vi "test_ResolveService_WithNewClusterId_RetriesAndSucceeds.vi"(8 "error in":errorcluster) -> (0 "error out":errorcluster, 2 "result":string, 3 "pass":bool)   [LabVIEW 2021, in "MeasurementServerTests.lvlib" / "Discovery Tests.lvlib"]
uses:
  Discovery Tests.lvlib
  Runtime/Clients/Discovery V1/NI Discovery V1 Client.lvlib
  MeasurementServerTests.lvlib
  gRPC/Generated APIs/ni/measurementlink/discovery/v1/RPC Messages/ni_measurementlink_discovery_v1_ResolveServiceRequest.ctl
  gRPC/Generated APIs/ni/measurementlink/discovery/v1/ni.measurementlink.discovery.v1.api.lvlib
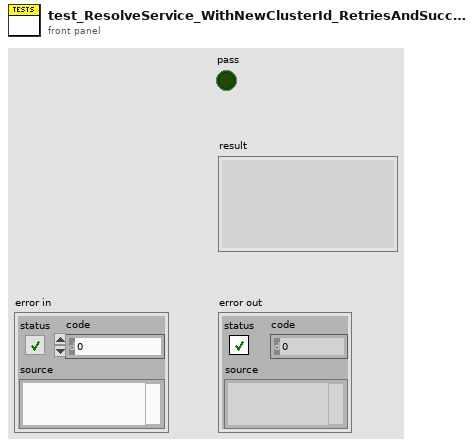
[diagram p1: front panel]
types:
  T1 = typedef "ni.measurementlink.discovery.v1.api.lvlib/ni_measurementlink_discovery_v1_ResolveServiceRequest.ctl" = cluster{"provided_interface":string, "service_class":string, "deployment_target":string, "version":string}
  T2 = typedef "ni.measurementlink.discovery.v1.api.lvlib/ni_measurementlink_discovery_v1_ServiceLocation.ctl" = cluster{"location":string, "insecure_port":string, "ssl_authenticated_port":string}
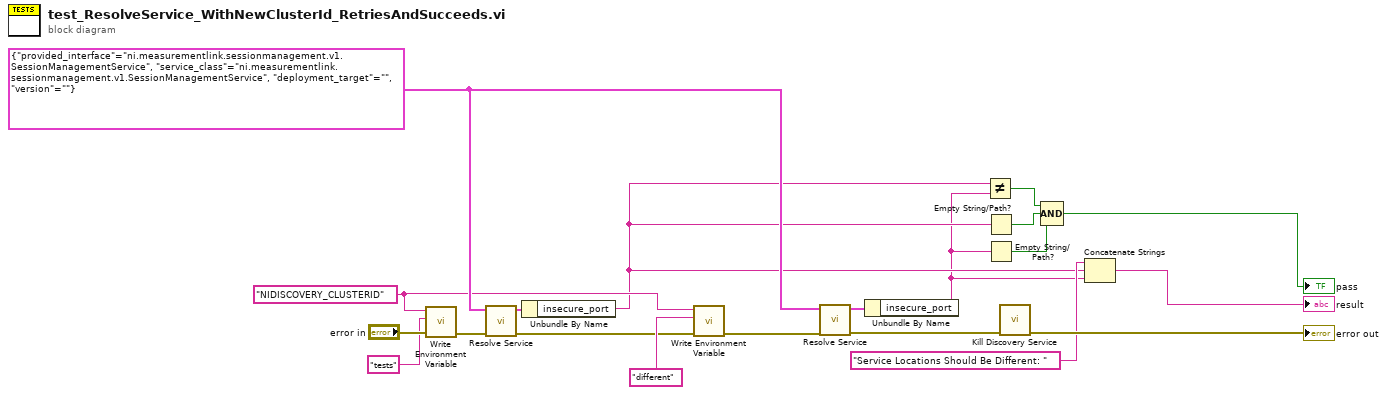
[diagram p0: block diagram]
diagram:
  w13 = "NIDISCOVERY_CLUSTERID" ("name")
  w17 = T1 {"provided_interface"="ni.measurementlink.sessionmanagement.v1.SessionManagementService", "service_class"="ni.measurementlink.sessionmanagement.v1.SessionManagementService", "deployment_target"="", "version"=""} ("request data")
  n1 = call "Write Environment Variable.vi"("error in"="error in", "value"="tests", "name"=w13) -> ("error out"=w16:errorcluster)  [unwired: 8 in]
  n2 = call "Resolve Service.vi"("error in"=w16, "request data"=w17) -> ("error out"=w15:errorcluster, "response data"=w9:T2)  [unwired: 8 in]
  n3 = Unbundle By Name(w9) -> ("insecure_port"=w3:string)
  n4 = call "Write Environment Variable.vi"("error in"=w15, "value"="different", "name"=w13) -> ("error out"=w14:errorcluster)  [unwired: 8 in]
  n5 = call "Resolve Service.vi"("error in"=w14, "request data"=w17) -> ("error out"=w12:errorcluster, "response data"=w10:T2)  [unwired: 8 in]
  n6 = Unbundle By Name(w10) -> ("insecure_port"=w2:string)
  n7 = Not Equal?(x=w3, y=w2) -> (x != y?=w8:bool)
  n8 = Empty String/Path?(string/path=w3) -> (empty?=w7:bool)
  n9 = Empty String/Path?(string/path=w2) -> (empty?=w6:bool)
  n10 = call "Kill Discovery Service.vi"("error in"=w12) -> ("error out"=→"error out":errorcluster)  [unwired: 10 in]
  n11 = Compound Arithmetic op=AND(w8, w7, w6) -> (→"pass":bool)
  n12 = Concatenate Strings("Service Locations Should Be Different: " ("string"), w3, w2) -> (→"result":string)
